vi "Write Settings.vi"(8 "error in (no error)":errorcluster, 10 "Settings":T1={"Serial Port for strømforsyning"="COM12", "Serial Port for SSI Interface"="COM12"}, 11 "ProgramSettings in":refnum<class "ProgramSettings.lvclass">) -> (0 "error out":errorcluster, 3 "ProgramSettings out":refnum<class "ProgramSettings.lvclass">)   [LabVIEW 2019, in "ProgramSettings.lvclass"]
uses:
  ProgramSettings.lvclass
  TypeDef/SettingParams.ctl
  ProgramSettings.lvclass/ProgramSettings.ctl
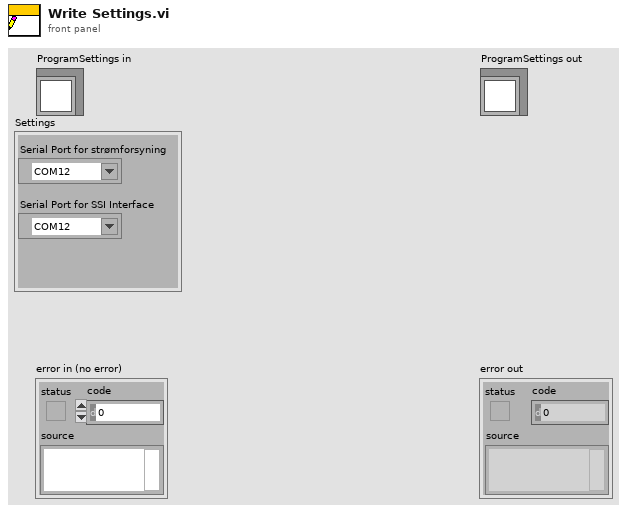
[diagram p1: front panel]
types:
  T1 = typedef "ProgramSettings.lvclass/SettingParams.ctl" = cluster{"Serial Port for strømforsyning":refnum<visa-resource-name>, "Serial Port for SSI Interface":refnum<visa-resource-name>}
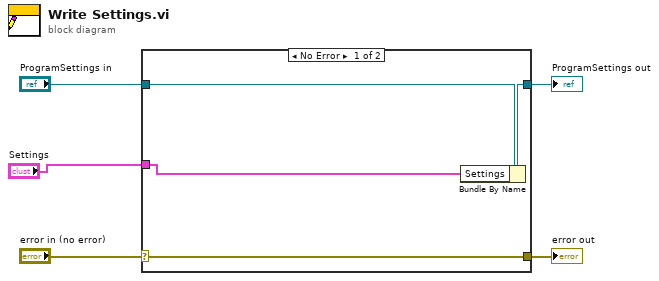
[diagram p0: block diagram]
diagram:
  n1 = case shown="No Error" "error in (no error)" {
    selector: "error in (no error)" -> [w9 w10]
    tunnel: [w9 w10] -> w4
    tunnel: [w7 w11] -> w2
    tunnel: "ProgramSettings in" -> [w8 w11]
    tunnel: "Settings" -> [w6 _]
    frame No Error {
      n2 = Bundle By Name(cluster=w8, "Settings"=w6) -> (w7:refnum<class "ProgramSettings.lvclass">)
    }
    frame Error {
    }
  }
  "error out" <- w4
  "ProgramSettings out" <- w2
